vi "MultiRegionData.vi"(0 "Action":T1(ring), 1 "Array No.":u32, 2 "Array Size / Index":u32, 3 "Data IN":dbl format="%.2f", 4 "Array IN":dbl[](array[numeric]), 5 "Region index":u16) -> (6 "Data OUT":dbl format="%.2f", 7 "Array OUT":dbl[](array[numeric]) format="%.2f")   [LabVIEW 2018]
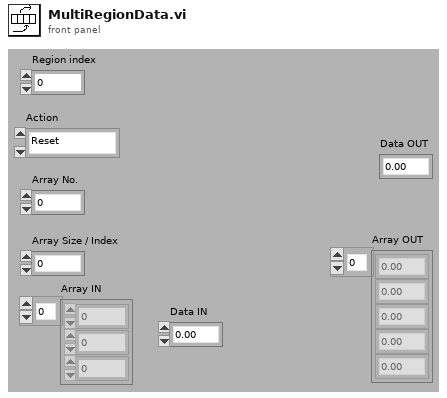
[diagram p1: front panel]
types:
  T1 = enum16{"Reset", "Read Array", "Read Element", "Write Element", "Write Array", "Add Element", "Add Array"}
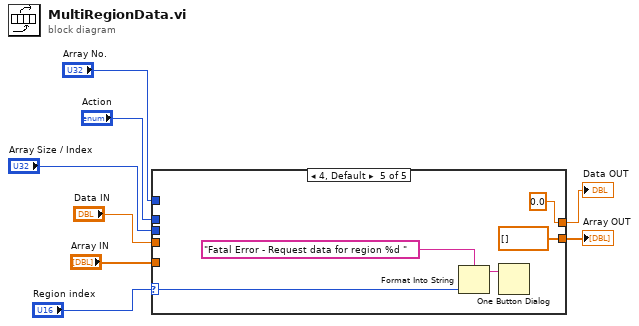
[diagram p0: block diagram]
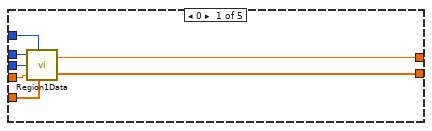
[diagram p2: hidden frame]
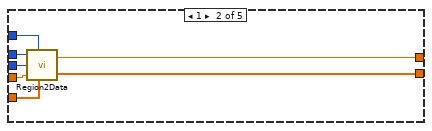
[diagram p3: hidden frame]
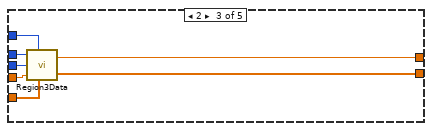
[diagram p4: hidden frame]
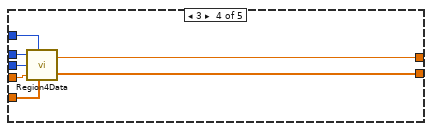
[diagram p5: hidden frame]
diagram:
  n1 = case shown="4, Default" "Region index" {
    selector: "Region index" -> [_ _ _ _ w37]
    tunnel: "Action" -> [w15 w22 w29 w36 _]
    tunnel: "Array No." -> [w14 w21 w28 w35 _]
    tunnel: "Array Size / Index" -> [w13 w20 w27 w34 _]
    tunnel: "Data IN" -> [w12 w19 w26 w33 _]
    tunnel: [w11 w18 w25 w32 0.0 ("Data OUT")] -> w1
    tunnel: [w10 w17 w24 w31 dbl[] [] ("Array OUT")] -> w5
    tunnel: "Array IN" -> [w9 w16 w23 w30 _]
    frame 0 {
      n2 = call "Region1Data.vi"("Action"=w15, "Array No."=w14, "Array Size / Index"=w13, "Data IN"=w12, "Array IN"=w9) -> ("Data OUT"=w11:dbl, "Array OUT"=w10:dbl[])
    }
    frame 1 {
      n3 = call "Region2Data.vi"("Action"=w22, "Array No."=w21, "Array Size / Index"=w20, "Data IN"=w19, "Array IN"=w16) -> ("Data OUT"=w18:dbl, "Array OUT"=w17:dbl[])
    }
    frame 2 {
      n4 = call "Region3Data.vi"("Action"=w29, "Array No."=w28, "Array Size / Index"=w27, "Data IN"=w26, "Array IN"=w23) -> ("Data OUT"=w25:dbl, "Array OUT"=w24:dbl[])
    }
    frame 3 {
      n5 = call "Region4Data.vi"("Action"=w36, "Array No."=w35, "Array Size / Index"=w34, "Data IN"=w33, "Array IN"=w30) -> ("Data OUT"=w32:dbl, "Array OUT"=w31:dbl[])
    }
    frame 4, Default {
      n6 = Format Into String(format string="Fatal Error - Request data for region %d " ("message"), w37) -> (resulting string=w38:string)  [unwired: 2 in, 1 out]
      n7 = One Button Dialog(message=w38) -> ()  [unwired: 1 in, 1 out]
    }
  }
  "Array OUT" <- w5
  "Data OUT" <- w1
